vi "Copy_UI_Data.vi"(8 "error in (no error)":errorcluster, 10 "IB_Source in":refnum<class "IB_Source.lvclass">, 11 "IB_TreeCtrFileItem.lvclass":refnum<class "IB_Tree_Item_Source_Contained_File.lvclass">) -> (0 "error out":errorcluster, 3 "IB_TreeCtrFileItem out":refnum<class "IB_Tree_Item_Source_Contained_File.lvclass">)   [LabVIEW 2020, in "IB_Tree_Item_Source_Contained_File.lvclass"]
uses:
  <vilib>/AppBuilder/IB_Classes/Tree_Item_Source_Contained_File/IB_Tree_Item_Source_Contained_File.lvclass
  <vilib>/AppBuilder/IB_Classes/Tree_Item_Source_Contained_File/IB_Tree_Item_Source_Contained_File.lvclass/IB_Tree_Item_Source_Contained_File.ctl
  <vilib>/AppBuilder/IB_Classes/Source/File/CtrFile/IB_CtrFile.lvclass
  <vilib>/AppBuilder/IB_Classes/Source/IB_Source.lvclass
  <vilib>/AppBuilder/IB_Classes/Tree_Item/IB_Tree_Item.lvclass
  e:/builds/penguin/labview/branches/2020/dev/dist/vi.lib/AppBuilder/IB_Classes/Tree_Item_Source_File/IB_Tree_Item_Source_File.lvclass
  e:/builds/penguin/labview/branches/2020/dev/dist/vi.lib/AppBuilder/IB_Classes/Tree_Item_Source/IB_Tree_Item_Source.lvclass
  e:/builds/penguin/labview/branches/2020/dev/dist/vi.lib/AppBuilder/IB_Classes/Tree_Item/IB_Tree_Item.lvclass
  e:/builds/penguin/labview/branches/2020/dev/dist/vi.lib/AppBuilder/IB_Classes/Tree_Item_Source_Contained_File/IB_Tree_Item_Source_Contained_File.lvclass
  e:/builds/penguin/labview/branches/2020/dev/dist/vi.lib/AppBuilder/IB_Classes/Source/File/IB_Source_File.lvclass
  e:/builds/penguin/labview/branches/2020/dev/dist/vi.lib/AppBuilder/IB_Classes/Source/IB_Source.lvclass
  e:/builds/penguin/labview/branches/2020/dev/dist/vi.lib/AppBuilder/IB_Classes/Source/File/CtrFile/IB_CtrFile.lvclass
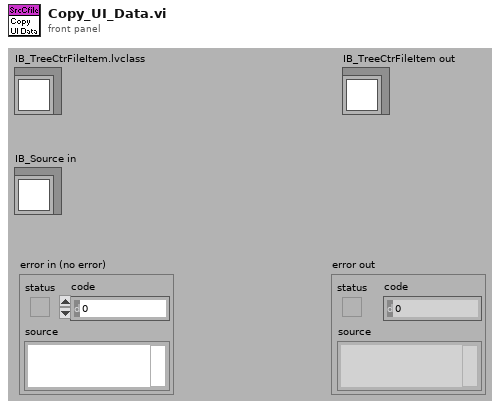
[diagram p1: front panel]
types:
  T1 = typedef "IB_CtrFile.ctl" = cluster{"parentTag":string, "force save?":bool}
  T2 = typedef "IB_Source.ctl" = cluster{"name":string, "sourceTag":string, "destTag":string, "path":path, "eng_installPath":string, "UI_inBuild?":bool, "str ref?":bool}
  T3 = typedef "IB_Tree_Item.ctl" = cluster{"symbol index":i32, "child tag":string, "parentTag":string, "left cell name":string}
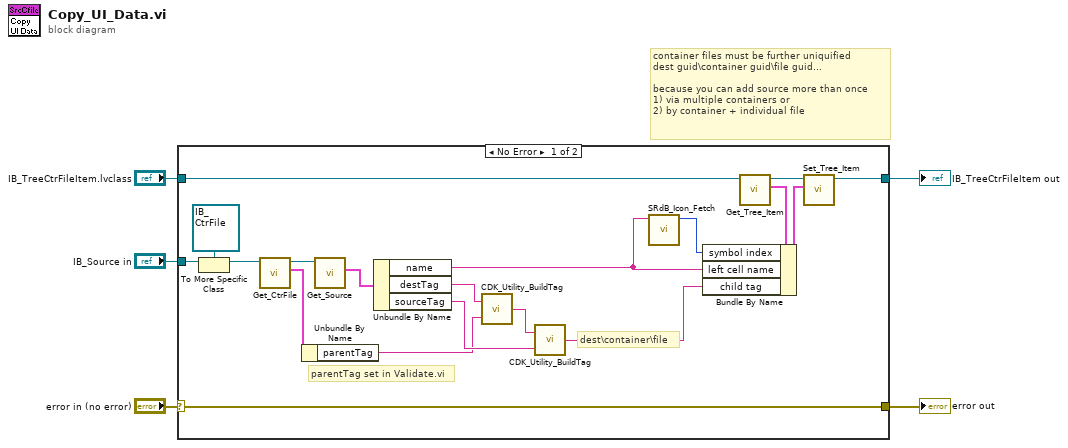
[diagram p0: block diagram]
diagram:
  # "container files must be further uniquified\ndest guid\\container guid\\file guid...\n\nbecause you can add source more than once\n1) via multiple containers or\n2) by container + individual file"
  n1 = case shown="No Error" "error in (no error)" {
    selector: "error in (no error)" -> [w11 w26]
    tunnel: "IB_Source in" -> [w22 _]
    tunnel: "IB_TreeCtrFileItem.lvclass" -> [w14 w25]
    tunnel: [w8 w25] -> w3
    tunnel: [w11 w26] -> w1
    frame No Error {
      # "parentTag set in Validate.vi"
      # "dest\\container\\file"
      n2 = To More Specific Class(target class=refnum<class "IB_CtrFile.lvclass"> refnum ("IB_CtrFile in"), reference=w22) -> (specific class reference=w23:refnum<class "IB_CtrFile.lvclass">)  [unwired: 1 in, 1 out]
      n3 = call <vilib>:"Get_CtrFile.vi"("IB_CtrFile in"=w23) -> ("parentTag"=w7:T1, "IB_CtrFile out"=w20:refnum<class "IB_CtrFile.lvclass">)  [unwired: 1 in, 8 out]
      n4 = Unbundle By Name(w7) -> ("parentTag"=w6:string)
      n5 = call <vilib>:"Get_Source.vi"("IB_Source in"=w20) -> ("data"=w21:T2)  [unwired: 1 in, 9 out]
      n6 = Unbundle By Name(w21) -> ("name"=w9:string, "destTag"=w19:string, "sourceTag"=w17:string)
      n7 = call <resource>:"CDK_Utility_BuildTag.vi"("name or relative path"=w6, "BasePath"=w19) -> ("appended path"=w18:string)
      n8 = call <resource>:"CDK_Utility_BuildTag.vi"("name or relative path"=w17, "BasePath"=w18) -> ("appended path"=w16:string)
      n9 = call <resource>:"SRdB_Icon_Fetch.vi"("filename"=w9) -> ("symbol index"=w10:i32)  [unwired: 1 in, 9 out]
      n10 = call <vilib>:"Get_Tree_Item.vi"("IB_TreeItem in"=w14) -> ("data"=w13:T3, "IB_TreeItem out"=w15:refnum<class "IB_Tree_Item_Source_Contained_File.lvclass">)  [unwired: 1 in, 8 out]
      n11 = Bundle By Name(cluster=w13, "symbol index"=w10, "left cell name"=w9, "child tag"=w16) -> (w12:T3)
      n12 = call <vilib>:"Set_Tree_Item.vi"("data"=w12, "IB_TreeItem in"=w15) -> ("IB_TreeItem out"=w8:refnum<class "IB_Tree_Item_Source_Contained_File.lvclass">)  [unwired: 1 in, 8 out]
    }
    frame Error {
    }
  }
  "IB_TreeCtrFileItem out" <- w3
  "error out" <- w1
